vi "Receive Config Data.vi"(8 "error in (no error)":errorcluster, 9 "Splitter":refnum<vi>, 10 "Config Data":T1, 11 "Message Log in":refnum<class "Message Log.lvclass">) -> (0 "error out":errorcluster, 3 "Message Log out":refnum<class "Message Log.lvclass">)   [LabVIEW 2017, in "Message Log.lvclass"]
uses:
  Message Log.lvclass
  C:/Program Files (x86)/National Instruments/LabVIEW 2017/vi.lib/addons/_Workers/Library/Classes/Worker/Worker.lvclass
  Config Data.ctl
  <vilib>/Utility/miscctls.llb/LVRectTypeDef.ctl
  <vilib>/addons/_Workers/Library/Classes/Worker/Worker.lvclass/Worker.ctl
  Message Log.lvclass/Message Log.ctl
  <vilib>/Utility/miscctls.llb/LVRowAndColumnTypeDef.ctl
  <vilib>/addons/_Workers/Library/Classes/Worker/Read MainVI Ref DVR.vi
  <vilib>/addons/_Workers/Library/Classes/Worker/Worker.lvclass
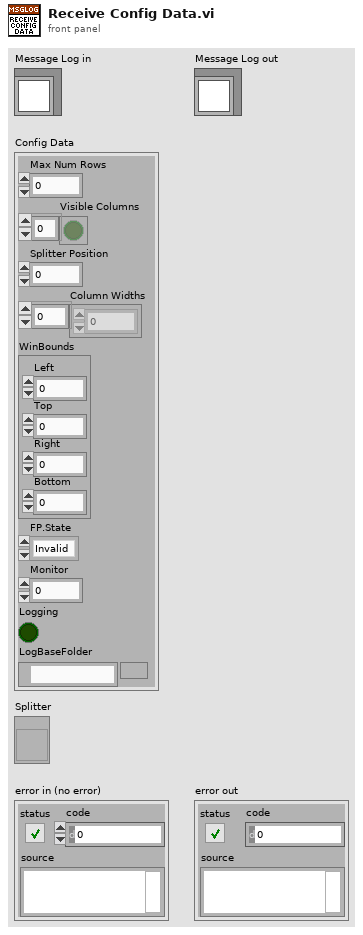
[diagram p1: front panel]
types:
  T1 = typedef "Message Log.lvclass/Config Data.ctl" = cluster{"Max Num Rows":i32, "Visible Columns":bool[], "Splitter Position":i32, "Column Widths":u32[], "WinBounds":T2, "FP.State":enum32{"Invalid", "Standard", "Closed", "Hidden", "Minimized", "Maximized"}, "Monitor":u16, "Logging":bool, "LogBaseFolder":path}
  T2 = typedef "LVRectTypeDef.ctl" = cluster{"Left":i16, "Top":i16, "Right":i16, "Bottom":i16}
  T3 = enum32{"Invalid", "Standard", "Closed", "Hidden", "Minimized", "Maximized"}
  T4 = typedef "LVRowAndColumnTypeDef.ctl" = cluster{"Row":i32, "Column":i32}
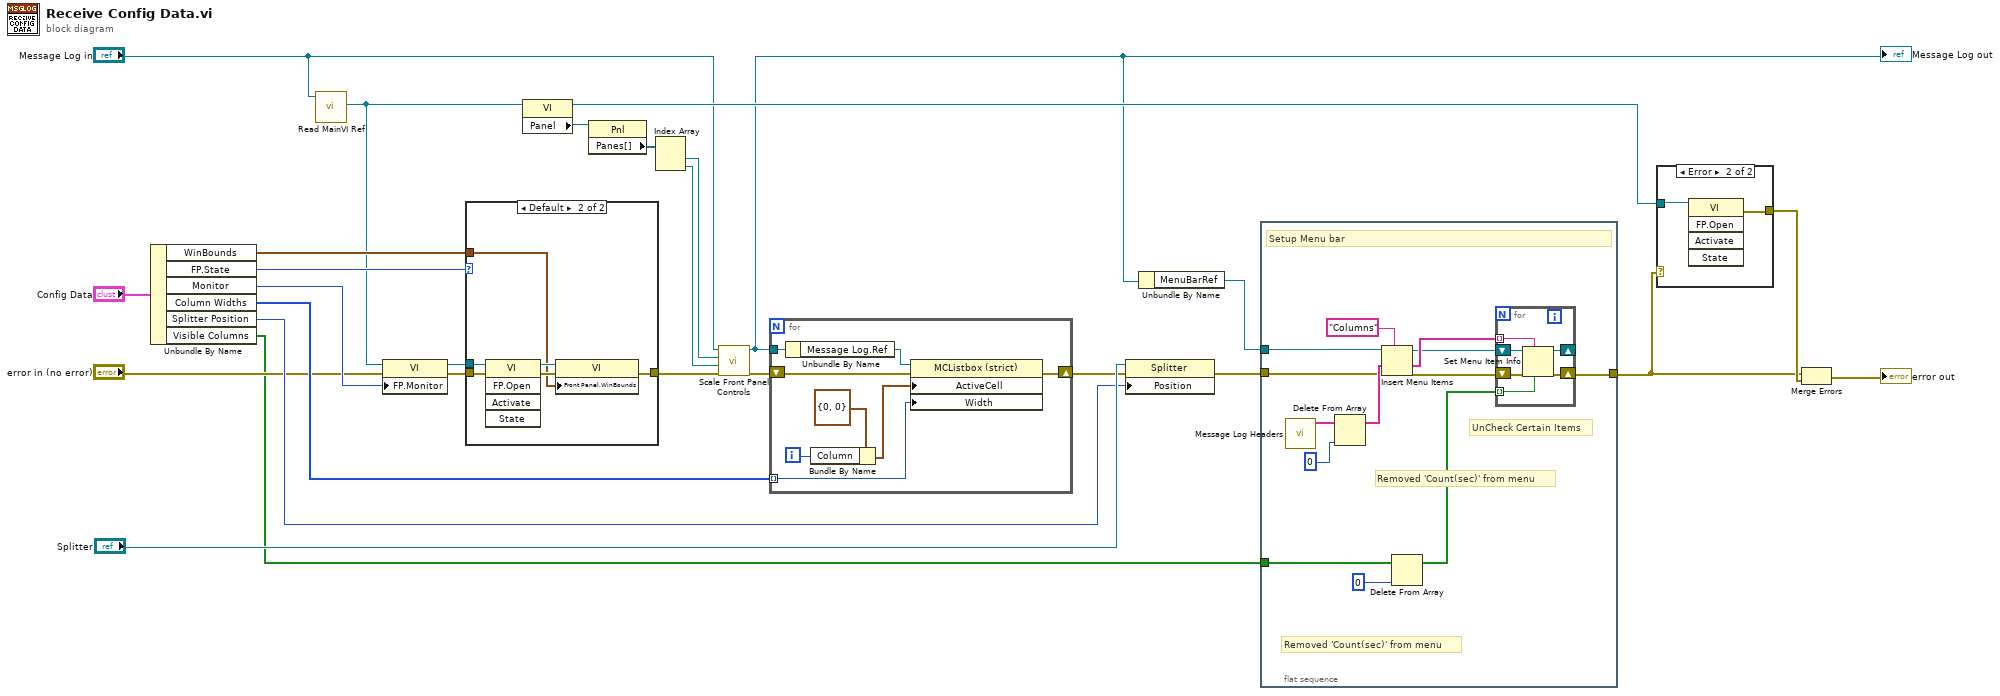
[diagram p0: block diagram]
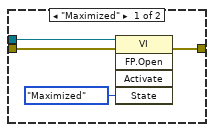
[diagram p3: hidden frame]
diagram:
  n1 = Unbundle By Name("Config Data") -> ("WinBounds"=w25:T2, "FP.State"=w26:T3, "Monitor"=w24:u16, "Column Widths"=w11:u32[], "Splitter Position"=w12:i32, "Visible Columns"=w4:bool[])
  n2 = call <vilib>:"Read MainVI Ref.vi"("Worker_"="Message Log in") -> ("MainVI Ref"=w8:refnum<vi>)  [unwired: 9 in, 1 out]
  n3 = property class="VI"(reference=w8, error in="error in (no error)", "FP.Monitor"=w24) -> (reference out=w23:refnum<vi>, error out=w22:errorcluster)
  n4 = case shown="Default" w26 {
    tunnel: [w31 w37] -> w27
    tunnel: w22 -> [w30 w36]
    tunnel: w23 -> [w29 w34]
    tunnel: w25 -> [_ w32]
    frame "Maximized" {
      n5 = invoke class="VI" method="FP.Open"(reference=w29, error in=w30, "State"=T3."Maximized" ("Front Panel Window:State")) -> (error out=w31:errorcluster)  [unwired: 2 in, 4 out]
    }
    frame Default {
      n6 = invoke class="VI" method="FP.Open"(reference=w34, error in=w36) -> (reference out=w33:refnum<vi>, error out=w35:errorcluster)  [unwired: 3 in, 3 out]
      n7 = property class="VI"(reference=w33, error in=w35, "Front Panel.WinBounds"=w32) -> (error out=w37:errorcluster)  [unwired: 1 out]
    }
  }
  n8 = property class="VI"(reference=w8) -> (reference out=w18:refnum<vi>, "Panel"=w21:refnum<vi>)  [unwired: 1 in, 1 out]
  n9 = property class="Pnl"(reference=w21) -> ("Panes[]"=w20:refnum<vi>[])  [unwired: 1 in, 2 out]
  n10 = Index Array(array=w20) -> (element #1=w19:refnum<vi>, element #2=w9:refnum<vi>)  [unwired: 2 in]
  n11 = call "Scale Front Panel Controls.vi"("error in (no error)"=w27, "Pane 2"=w9, "Pane"=w19, "Message Log in"="Message Log in") -> ("error out"=w14:errorcluster, "Message Log out"=w3:refnum<class "Message Log.lvclass">)  [unwired: 6 in]
  "Message Log out" <- w3
  n12 = for {
    shift-right: [w44] -> w7
    shift-left: w14 -> [w45]
    tunnel: w11 -> [w40] mode=indexing
    tunnel: w3 -> [w39]
    i -> [w42]
    n13 = Unbundle By Name(w39) -> ("Message Log.Ref"=w38:refnum<vi>)
    n14 = Bundle By Name(cluster=T4 {"Row"=0, "Column"=0} ("Active Cell:Active Cell"), "Column"=w42) -> (w41:T4)
    n15 = property class="MCListbox (strict)"(reference=w38, error in=w45, "ActiveCell"=w41, "Width"=w40) -> (error out=w44:errorcluster)  [unwired: 1 out]
  }
  n16 = property class="Splitter"(reference="Splitter", error in=w7, "Position"=w12) -> (error out=w6:errorcluster)  [unwired: 1 out]
  n17 = Unbundle By Name(w3) -> ("MenuBarRef"=w2:refnum<k9>)
  n18 = flat-sequence {
    tunnel: w6 -> [w49]
    tunnel: [w48] -> w5
    tunnel: w4 -> [w47]
    tunnel: w2 -> [w46]
    frame #0 {
      # "Removed 'Count(sec)' from menu"
      # "Removed 'Count(sec)' from menu"
      # "UnCheck Certain Items"
      # "Setup Menu bar"
      n19 = call "Message Log Headers.vi"() -> ("Message Log Headers"=w54:string[])  [unwired: 11 in]
      n20 = Delete From Array(array=w54, index=0) -> (array with subset deleted=w53:string[])  [unwired: 1 in, 1 out]
      n21 = Insert Menu Items(5:"Columns" ("L10n_menu tag"), 6:w49, 7:w53, 9:w46) -> (0:w57:errorcluster, 1:w56:string[], 3:w55:refnum<k9>)  [unwired: 2 in]
      n22 = Delete From Array(array=w47, index=0) -> (array with subset deleted=w50:bool[])  [unwired: 1 in, 1 out]
      n23 = for {
        tunnel: w56 -> [w63] mode=indexing
        shift-right: [w61] -> w48
        shift-left: w57 -> [w64]
        tunnel: w50 -> [w60] mode=indexing
        shift-right: [w59] -> _
        shift-left: w55 -> [w62]
        n24 = Set Menu Item Info(6:w60, 7:w63, 8:w64, 11:w62) -> (0:w61:errorcluster, 3:w59:refnum<k9>)  [unwired: 3 in]
      }
    }
  }
  n25 = case shown="Error" w5 {
    selector: w5 -> [w65 _]
    tunnel: [w65 w67] -> w16
    tunnel: w18 -> [_ w66]
    frame No Error {
    }
    frame Error {
      n26 = invoke class="VI" method="FP.Open"(reference=w66) -> (error out=w67:errorcluster)  [unwired: 4 in, 4 out]
    }
  }
  n27 = Merge Errors(w5, w16) -> (→"error out":errorcluster)
